vi "sortRows.vi"(11 "Array in":dbl[][](array[numeric])) -> (3 "Array out":dbl[][](array[numeric]))   [LabVIEW 2017]
doc: "Sort all rows in array"
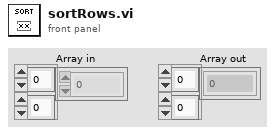
[diagram p1: front panel]
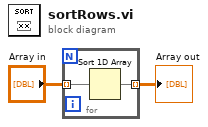
[diagram p0: block diagram]
diagram:
  n1 = for {
    tunnel: "Array in" -> [w4] mode=indexing
    tunnel: [w3] -> w2 mode=indexing
    n2 = Sort 1D Array(array=w4) -> (sorted array=w3:dbl[])
  }
  "Array out" <- w2
